vi "MccHat_init.vi"(8 "error in":errorcluster, 10 "port":u16, 11 "address":string) -> (0 "error out":errorcluster, 3 "conn_id":refnum<k5>, 4 "status":bool)   [LabVIEW 2019]
panel:
  out "status_each":bool[](array[boolean])
  out "msg_each":string[](array[string])
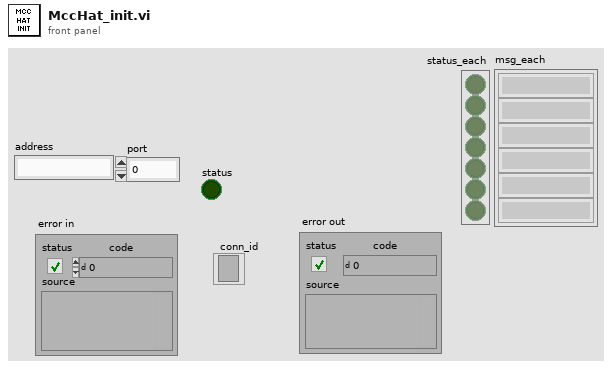
[diagram p1: front panel]
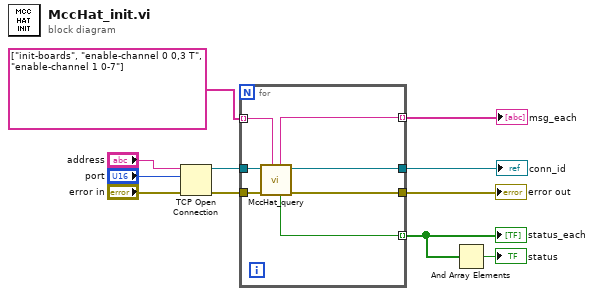
[diagram p0: block diagram]
diagram:
  n1 = TCP Open Connection(address="address", remote port or service name="port", error in (no error)="error in") -> (connection ID=w7:refnum<k5>, error out=w8:errorcluster)  [unwired: 2 in]
  n2 = for {
    tunnel: w8 -> [w18]
    tunnel: w7 -> [w17]
    tunnel: [w16] -> w4 mode=indexing
    tunnel: string[] ["init-boards", "enable-channel 0 0,3 T", "enable-channel 1 0-7"] -> [w15] mode=indexing
    tunnel: [w14] -> w5 mode=indexing
    tunnel: [w13] -> w2
    tunnel: [w12] -> w1
    n3 = call "MccHat_query.vi"("command"=w15, "error in"=w18, "conn_id_in"=w17) -> ("error out"=w13:errorcluster, "conn_id_out"=w12:refnum<k5>, "status"=w16:bool, "string_raw"=w14:string)  [unwired: 4 in, 1 out]
  }
  "error out" <- w2
  "msg_each" <- w5
  "conn_id" <- w1
  "status_each" <- w4
  n4 = And Array Elements(Boolean array=w4) -> (logical AND=→"status":bool)
